vi "Get Source Path From Install Path.vi"(8 "Error In":errorcluster, 10 "Install File Path":path, 11 "Configuration":T1) -> (0 "Error Out":errorcluster, 1 "Source File Path":path, 2 "Install File Path":path, 3 "Configuraiton":T1)   [LabVIEW 2011, in "LVH-Build-Tools.lvlib"]
doc: "Get the source path of a file based on its install path.\n\nThis VI strips the install root path from the file path and prepends the source path."
uses:
  LVH-Build-Tools.lvlib
  Type Defs/Configuration.ctl
  Type Defs/Install Configuration.ctl
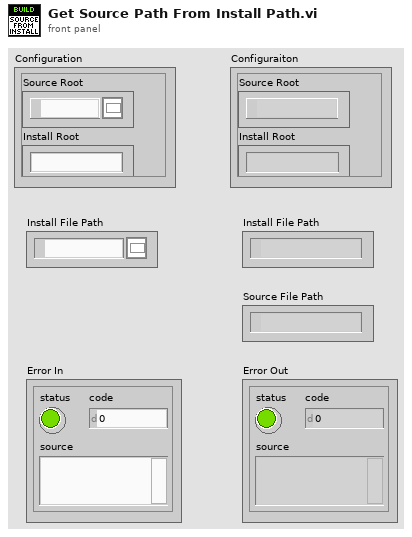
[diagram p1: front panel]
types:
  T1 = typedef "LVH-Build-Tools.lvlib/Configuration.ctl" = cluster{"Source Root":path, "Install Root":string, "Components":string[], "Ignore":string[], "Config Files":path[], "LV Directories":path[], "Install Paths":T2}
  T2 = typedef "LVH-Build-Tools.lvlib/Install Configuration.ctl" = cluster{"LabVIEW Directory":path, "Project Source Config":path}
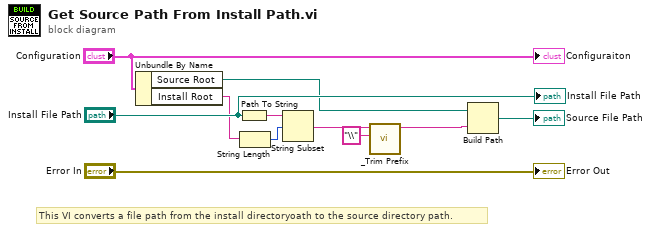
[diagram p0: block diagram]
diagram:
  # "This VI converts a file path from the install directoryoath to the source directory path."
  n1 = Unbundle By Name("Configuration") -> ("Source Root"=w5:path, "Install Root"=w7:string)
  n2 = Path To String(path="Install File Path") -> (string=w10:string)
  n3 = String Length(string=w7) -> (length=w11:i32)
  n4 = String Subset(string=w10, offset (0)=w11) -> (substring=w3:string)  [unwired: 1 in]
  n5 = call "_Trim Prefix.vi"("Prefix"="\\", "String"=w3) -> ("String"=w2:string)  [unwired: 9 in]
  n6 = Build Path(base path=w5, name or relative path=w2) -> (appended path=→"Source File Path":path)
  "Error Out" <- "Error In"
  "Configuraiton" <- "Configuration"
  "Install File Path" <- "Install File Path"
